vi "test-discretization-15.vi"(8 "error in (no error)":errorcluster) -> (0 "error out":errorcluster, 3 "All Tests Passed":bool)   [LabVIEW 2019]
uses:
  <vilib>/Analysis/Matrix/Datatypes/ComplexMatrix.ctl
  <vilib>/Analysis/Matrix/Datatypes/RealMatrix.ctl
  <vilib>/Analysis/7linalg.llb/Eigenvalue and Vectors Output Option.ctl
  <vilib>/Rock Robotics/WPI/ThirdParty/JAS_Junk/TrajLib/MatBuilder_Create.vi
  <vilib>/Rock Robotics/WPI/ThirdParty/JAS_Junk/TrajLib/MatrixHelper_CoerceSize.vi
  <vilib>/Rock Robotics/WPI/ThirdParty/JAS_Junk/TrajLib/Matrix_Transpose.vi
  <vilib>/Rock Robotics/WPI/ThirdParty/JAS_Junk/TrajLib/Matrix_AssignBlock.vi
  <vilib>/Rock Robotics/WPI/ThirdParty/JAS_Junk/TrajLib/Matrix_Exp.vi
  <vilib>/Rock Robotics/WPI/ThirdParty/JAS_Junk/TrajLib/Matrix_Block.vi
  <vilib>/Analysis/baseanly.llb/A x B.vi
  <vilib>/Analysis/baseanly.llb/Real A x B.vi
  <vilib>/Analysis/7linalg.llb/Transpose Matrix.vi
  <vilib>/Analysis/7linalg.llb/Real Transpose Matrix.vi
  <vilib>/Analysis/_algsub.llb/Matrix Norm.vi
  <vilib>/Analysis/_algsub.llb/Real Matrix Norm.vi
  <vilib>/Analysis/7linalg.llb/Matrix Exp.vi
  <vilib>/Analysis/7linalg.llb/Real Matrix Exp.vi
  <vilib>/Analysis/7linalg.llb/Real Eigenvalues and Vectors.vi
  <vilib>/Analysis/Matrix/Numeric/Multiply/Multiply.vi
  <vilib>/Analysis/Matrix/Numeric/Multiply/Multiply - RM,R.vi
  <vilib>/Analysis/Matrix/Numeric/Add/Add.vi
  <vilib>/Analysis/Matrix/Numeric/Add/Add - RM,RM.vi
  <vilib>/Analysis/Matrix/Numeric/Subtract/Subtract - RM,RM.vi
  <vilib>/Rock Robotics/WPI/ThirdParty/JAS_Junk/TrajLib/Trajectory_Library.lvlib
  <vilib>/Analysis/NI_AALPro.lvlib
  <vilib>/Analysis/Matrix/NI_Matrix.lvlib
panel:
  out "DiscA Taylor":T1
  out "DiscQ Taylor":T1
  out "DiscQ-NormF":dbl format="%.4f"
  out "Eigenvalues 2":cdb[](array[numeric])
  out "Pos Semidefiniate 2":bool
  out "error 2":i32
  out "ApproxEquals 2":bool
  out "ApproxEquals":bool
  out "DiscQ Taylor\nNOT":T1
  out "DiscA Taylor\nNOT":T1
  out "Error 2":bool
  out "DiscA":T1
  out "DiscQ Int":T1
  in  "Cluster":cluster{"ContQ":T1, "ContA":T1}
  out "int discq":bool
  out "Pos Semidefiniate":bool
  out "Eigenvectors":T2
  out "error":i32
  out "Eigenvalues":cdb[](array[numeric])
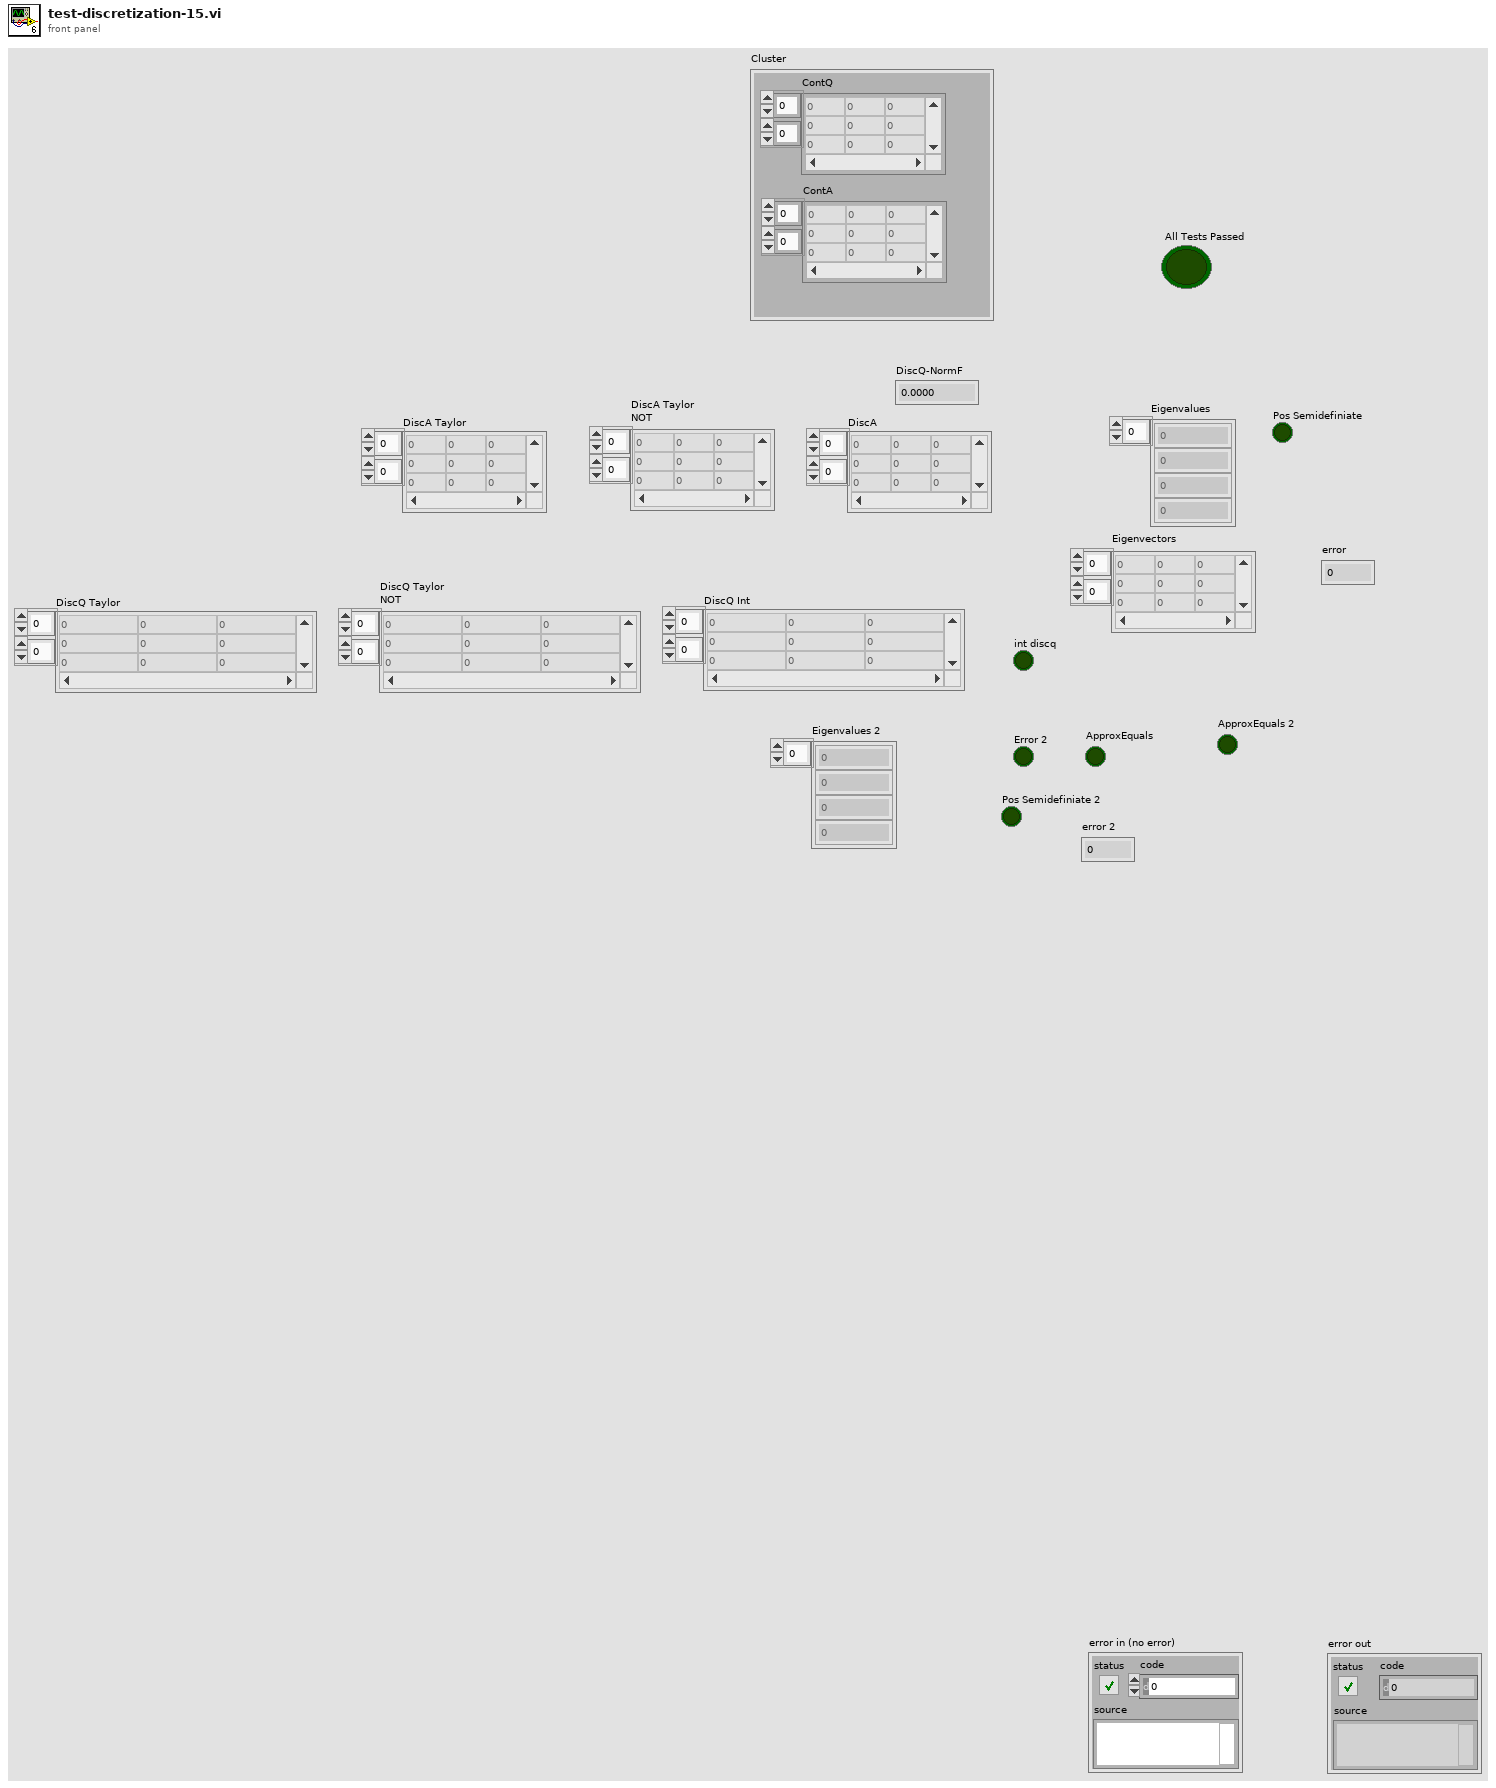
[diagram p1: front panel]
types:
  T1 = typedef "NI_Matrix.lvlib/RealMatrix.ctl" = dbl[][]
  T2 = typedef "NI_Matrix.lvlib/ComplexMatrix.ctl" = cdb[][]
  T3 = typedef "NI_AALPro.lvlib/Eigenvalue and Vectors Output Option.ctl" = i32
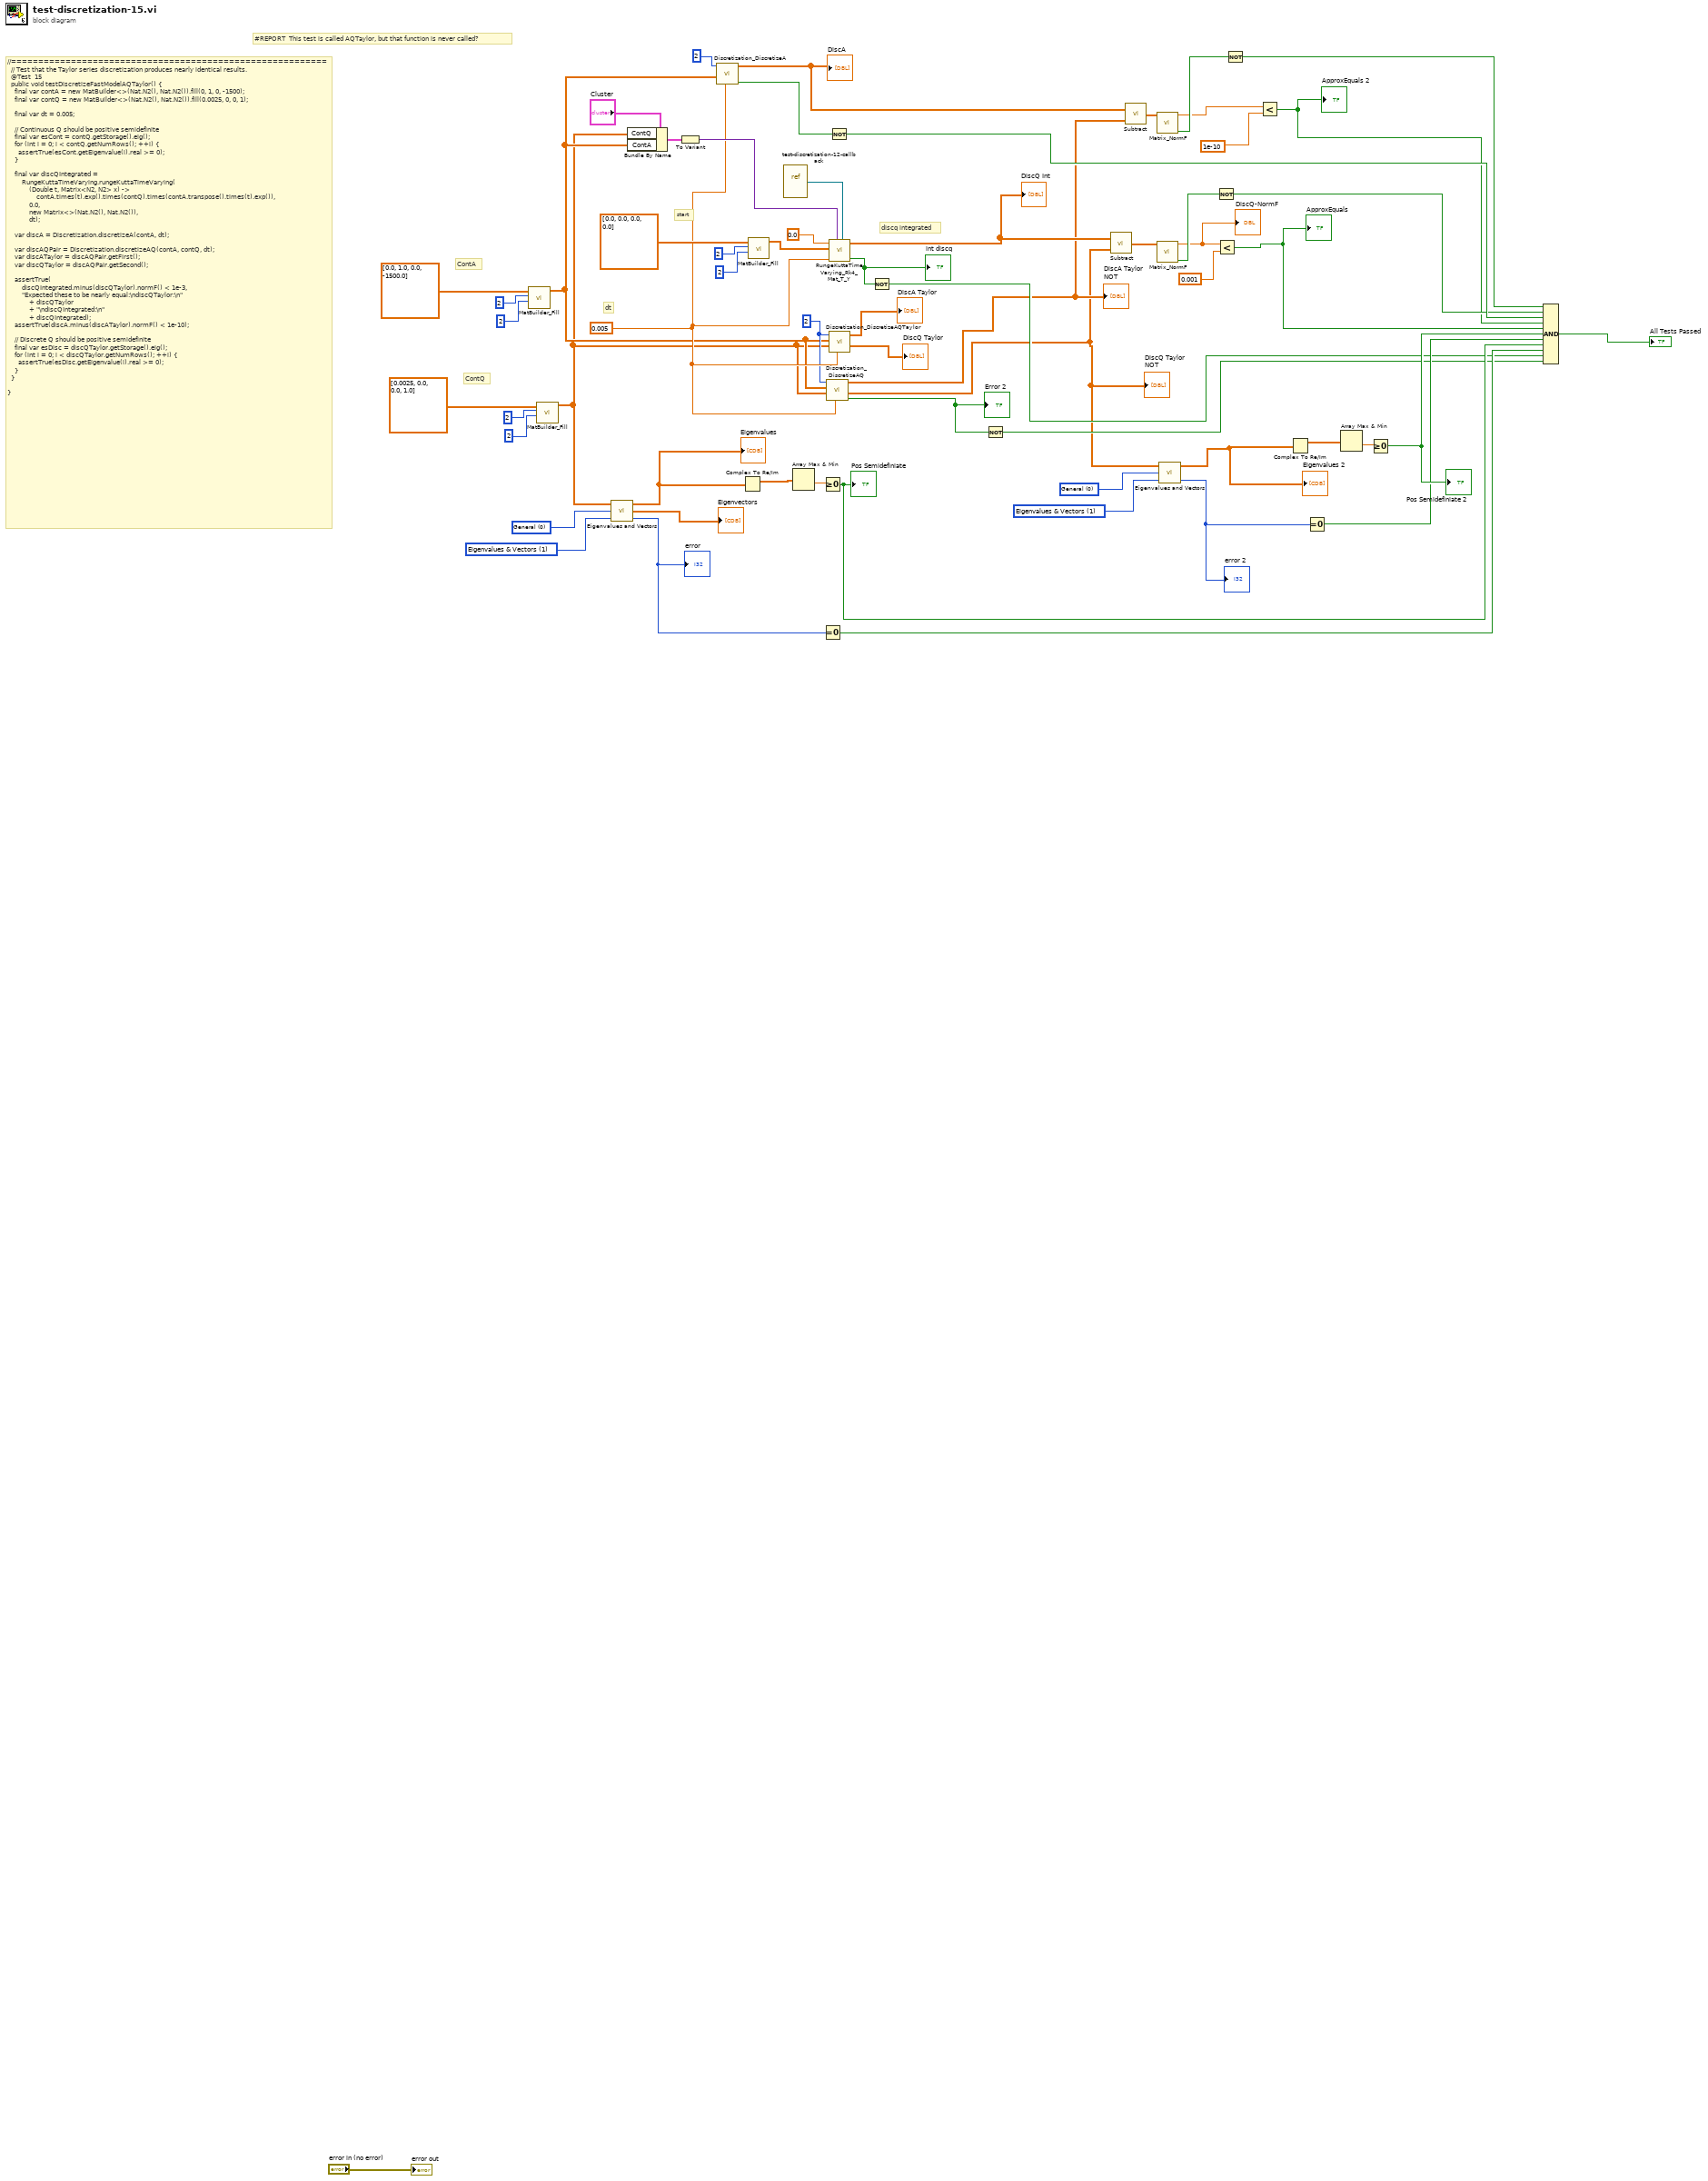
[diagram p0: block diagram]
diagram:
  w29 = T3 1 items=["Eigenvalues", "Eigenvalues & Vectors"] ("output option")
  w30 = 0 items=["General", "Symmetric"] ("matrix type")
  w37 = 2 ("States")
  w38 = 0.005 ("dT_Seconds")
  w55 = T3 1 items=["Eigenvalues", "Eigenvalues & Vectors"] ("output option")
  w56 = 0 items=["General", "Symmetric"] ("matrix type")
  # "#REPORT  This test is called AQTaylor, but that function is never called?"
  # "dt"
  # "discq integrated"
  # "start"
  # "ContQ"
  # "ContA"
  # "//==========================================================\n  // Test that the Taylor series discretization produces nearly identical results.\n  @Test  15\n  public void testDiscretizeFastModelAQTaylor() {\n    final var contA = new MatBuilder<>(Nat.N2(), Nat.N2()).fill(0, 1, 0, -1500);\n    final var contQ = new MatBuilder<>(Nat.N2(), Nat.N2()).fill(0.0025, 0, 0, 1);\n\n    final var dt = 0.005;\n\n    // Continuous Q should be positive semidefinite\n    final var esCont = contQ.getStorage().eig();\n    for (int i = 0; i < contQ.getNumRows(); ++i) {\n      assertTrue(esCont.getEigenvalue(i).real >= 0);\n    }\n\n    final var discQIntegrated =\n        RungeKuttaTimeVarying.rungeKuttaTimeVarying(\n            (Double t, Matrix<N2, N2> x) ->\n                contA.times(t).exp().times(contQ).times(contA.transpose().times(t).exp()),\n            0.0,\n            new Matrix<>(Nat.N2(), Nat.N2()),\n            dt);\n\n    var discA = Discretization.discretizeA(contA, dt);\n\n    var discAQPair = Discretization.discretizeAQ(contA, contQ, dt);\n    var discATaylor = discAQPair.getFirst();\n    var discQTaylor = discAQPair.getSecond();\n\n    assertTrue(\n        discQIntegrated.minus(discQTaylor).normF() < 1e-3,\n        \"Expected these to be nearly equal:\\ndiscQTaylor:\\n\"\n            + discQTaylor\n            + \"\\ndiscQIntegrated:\\n\"\n            + discQIntegrated);\n    assertTrue(discA.minus(discATaylor).normF() < 1e-10);\n\n    // Discrete Q should be positive semidefinite\n    final var esDisc = discQTaylor.getStorage().eig();\n    for (int i = 0; i < discQTaylor.getNumRows(); ++i) {\n      assertTrue(esDisc.getEigenvalue(i).real >= 0);\n    }\n  }\n\n}"
  n1 = call <vilib>:"MatBuilder_Fill.vi"("Columns"=2, "Rows"=2, "Value List"=dbl[] [0.0, 1.0, 0.0, -1500.0]) -> ("output matrix"=w36:T1)  [unwired: 8 in]
  n2 = call <vilib>:"MatBuilder_Fill.vi"("Columns"=2, "Rows"=2, "Value List"=dbl[] [0.0025, 0.0, 0.0, 1.0]) -> ("output matrix"=w35:T1)  [unwired: 8 in]
  n3 = call-poly <vilib>:"Eigenvalues and Vectors.vi"("output option"=w55, "matrix type"=w56, "Input Matrix"=w35) -> ("error"=w21:i32, "Eigenvectors"=→"Eigenvectors":T2, "Eigenvalues"=w52:cdb[])
  "Eigenvalues" <- w52
  "error" <- w21
  n4 = Bundle By Name(cluster="Cluster", "ContQ"=w35, "ContA"=w36) -> (w42:cluster{"ContQ":T1, "ContA":T1})
  n5 = To Variant(anything=w42) -> (Variant=w41:variant)
  n6 = call <vilib>:"Discretization_DiscretizeA.vi"("dT_Seconds"=w38, "ContA"=w36, "States"=2) -> ("Error"=w17:bool, "DiscA"=w31:T1)  [unwired: 7 in]
  "DiscA" <- w31
  n7 = Complex To Re/Im(x + iy=w52) -> (x=w51:dbl[])  [unwired: 1 out]
  n8 = call <vilib>:"MatBuilder_Fill.vi"("Columns"=2, "Rows"=2, "Value List"=dbl[] [0.0, 0.0, 0.0, 0.0]) -> ("output matrix"=w44:T1)  [unwired: 8 in]
  n9 = vi-ref "test-discretization-12-callback.vi"() -> (w49:refnum<vi>)
  n10 = Array Max & Min(array=w51) -> (min value=w50:dbl)  [unwired: 3 out]
  n11 = Greater Or Equal To 0?(x=w50) -> (x >= 0?=w22:bool)
  "Pos Semidefiniate" <- w22
  n12 = Equal To 0?(x=w21) -> (x = 0?=w20:bool)
  n13 = call <vilib>:"Discretization_DiscretizeAQ.vi"("dT_Seconds"=w38, "ContQ"=w35, "ContA"=w36, "States"=w37) -> ("Error"=w11:bool, "DiscQ"=w9:T1, "DiscA"=w10:T1)  [unwired: 5 in]
  "Error 2" <- w11
  "DiscA Taylor\nNOT" <- w10
  "DiscQ Taylor\nNOT" <- w9
  n14 = Not(x=w17) -> (.not. x?=w16:bool)
  n15 = call <vilib>:"RungeKuttaTimeVarying_Rk4_Mat_T_Y.vi"("Func_T_Y_Extra"=w49, "PassedData"=w41, "dT_Seconds"=w38, "Y"=w44, "T"=0.0) -> ("Error"=w40:bool, "OUTPUT"=w34:T1)  [unwired: 5 in]
  "int discq" <- w40
  "DiscQ Int" <- w34
  n16 = call <vilib>:"Discretization_DiscretizeAQTaylor.vi"("dT_Seconds"=w38, "ContQ"=w35, "ContA"=w36, "States"=w37) -> ("DiscQ"=→"DiscQ Taylor":T1, "DiscA"=→"DiscA Taylor":T1)  [unwired: 5 in, 1 out]
  n17 = Not(x=w40) -> (.not. x?=w18:bool)
  n18 = Not(x=w11) -> (.not. x?=w19:bool)
  n19 = call-poly <vilib>:"Subtract.vi"("Real Matrix B"=w9, "Real Matrix A"=w34) -> ("A - B"=w33:T1)
  n20 = call-poly <vilib>:"Subtract.vi"("Real Matrix B"=w10, "Real Matrix A"=w31) -> ("A - B"=w32:T1)
  n21 = call <vilib>:"Matrix_NormF.vi"("input matrix"=w32) -> ("Error"=w15:bool, "normF"=w5:dbl)  [unwired: 9 in]
  n22 = call <vilib>:"Matrix_NormF.vi"("input matrix"=w33) -> ("Error"=w14:bool, "normF"=w8:dbl)  [unwired: 9 in]
  "DiscQ-NormF" <- w8
  n23 = call-poly <vilib>:"Eigenvalues and Vectors.vi"("output option"=w29, "matrix type"=w30, "Input Matrix"=w9) -> ("error"=w24:i32, "Eigenvalues"=w28:cdb[])  [unwired: 1 out]
  "error 2" <- w24
  "Eigenvalues 2" <- w28
  n24 = Not(x=w14) -> (.not. x?=w13:bool)
  n25 = Less?(x=w8, y=0.001) -> (x < y?=w6:bool)
  "ApproxEquals" <- w6
  n26 = Not(x=w15) -> (.not. x?=w12:bool)
  n27 = Less?(x=w5, y=1e-10 ("Tolerance")) -> (x < y?=w4:bool)
  "ApproxEquals 2" <- w4
  n28 = Complex To Re/Im(x + iy=w28) -> (x=w27:dbl[])  [unwired: 1 out]
  n29 = Equal To 0?(x=w24) -> (x = 0?=w23:bool)
  n30 = Array Max & Min(array=w27) -> (min value=w26:dbl)  [unwired: 3 out]
  n31 = Greater Or Equal To 0?(x=w26) -> (x >= 0?=w25:bool)
  "Pos Semidefiniate 2" <- w25
  n32 = Compound Arithmetic op=AND(w12, w13, w16, w4, w6, w25, w23, w22, w20, w18, w19) -> (→"All Tests Passed":bool)
  "error out" <- "error in (no error)"
